vi "SV RMS Average Spectra (Complex).vi"(0 "complex spectra":T7(array[cluster]) {"spectrum info"."x-axis units" items=["Time (s)"=0, "Frequency-CB (Hz)"=1, "Frequency-CPB (Hz)"=1248, "Frequency-Arbitrary (Hz)"=2357, "Quefrency (s)"=2, "Revolutions (rev)"=3, "Order"=4, "Speed (RPM)"=11, "Speed (rad/s)"=21, "Index"=65535]; "spectrum info"."weighting filter" items=["Linear", "A-weighting", "B-weighting", "C-weighting", "ITU-R 468-4", "Dolby", "CCITT", "C-message", "Wb", "Wc", "Wd", "We", "Wf", "Wh", "Wj", "Wk", "Wm", "AES17 20 kHz lowpass", "AES17 40 kHz lowpass", "AES17 20 kHz highpass", "AES17 40 kHz highpass"]; "spectrum info"."dB reference [EU]" format="%.2f"; "spectrum info"."engineering units" items=["custom..."=0, "V"=1, "A"=21, "C"=30, "pC"=31, "s"=32, "-"=29, "Pa"=2, "N"=20, "g"=3, "m/s^2"=4, "m/s"=5, "m"=6, "mm/s"=12, "mm"=13, "micron/s"=14, "micron"=15, "in/s^2"=7, "in/s"=8, "in"=9, "mil/s"=10, "mil"=11, "rad/s^2"=16, "rad/s"=17, "rad"=18, "deg/s^2"=26, "deg/s"=27, "deg"=28, "RPM"=22, "cycle/s^2"=23, "Hz"=24, "cycle"=25, "strain"=19]; "spectrum info"."spectral info"."window" items=["None "=0, "Hanning"=1, "Hamming"=2, "Blackman-Harris"=3, "Exact Blackman"=4, "Blackman"=5, "Flat Top"=6, "4 Term B-Harris "=7, "7 Term B-Harris"=8, "Low Sidelobe"=9, "Force - Exponential"=10, "Gaussian"=62]; "complex spectrum response"."complex spectrum" format="%.2f"; "complex spectrum response"."df" format="%.2f"; "complex spectrum response"."f0" format="%.2f"}, 5 "error in (no error)":errorcluster) -> (13 "averages completed":dbl, 14 "rms average spectrum":cluster{"f0":dbl, "df":dbl, "magnitude":dbl[]} {"magnitude" format="%.2p"; "df" format="%.2p"; "f0" format="%.2p"}, 18 "spectrum info":T1={"channel name"="", "description"="", "x-axis units"=0, "spectral info"={"spectrum type"=enum."Power [Magnitude^2]", "linear/dB"=enum."linear", "window"=0, "window size"=0, "FFT size"=0}, "engineering units"=1, "custom label"="", "dB reference [EU]"=0.0, "peak units"=enum."rms", "weighting filter"=0, "spectral density?"=FALSE, "unit label"="", "spectrum skewed?"=FALSE, "complimentary spectrum units"=enum."none"} {"x-axis units" items=["Time (s)"=0, "Frequency-CB (Hz)"=1, "Frequency-CPB (Hz)"=1248, "Frequency-Arbitrary (Hz)"=2357, "Quefrency (s)"=2, "Revolutions (rev)"=3, "Order"=4, "Speed (RPM)"=11, "Speed (rad/s)"=21, "Index"=65535]; "weighting filter" items=["Linear", "A-weighting", "B-weighting", "C-weighting", "ITU-R 468-4", "Dolby", "CCITT", "C-message", "Wb", "Wc", "Wd", "We", "Wf", "Wh", "Wj", "Wk", "Wm", "AES17 20 kHz lowpass", "AES17 40 kHz lowpass", "AES17 20 kHz highpass", "AES17 40 kHz highpass"]; "dB reference [EU]" format="%.2f"; "engineering units" items=["custom..."=0, "V"=1, "A"=21, "C"=30, "pC"=31, "s"=32, "-"=29, "Pa"=2, "N"=20, "g"=3, "m/s^2"=4, "m/s"=5, "m"=6, "mm/s"=12, "mm"=13, "micron/s"=14, "micron"=15, "in/s^2"=7, "in/s"=8, "in"=9, "mil/s"=10, "mil"=11, "rad/s^2"=16, "rad/s"=17, "rad"=18, "deg/s^2"=26, "deg/s"=27, "deg"=28, "RPM"=22, "cycle/s^2"=23, "Hz"=24, "cycle"=25, "strain"=19]; "spectral info"."window" items=["None "=0, "Hanning"=1, "Hamming"=2, "Blackman-Harris"=3, "Exact Blackman"=4, "Blackman"=5, "Flat Top"=6, "4 Term B-Harris "=7, "7 Term B-Harris"=8, "Low Sidelobe"=9, "Force - Exponential"=10, "Gaussian"=62]}, 19 "error out":errorcluster)   [LabVIEW 2017]
doc: "Computes the linear RMS-averaged power spectrum of <B>scaled signal [EU]</B> in a linear scale. Use the power spectrum to quantify signal components as a function of frequency. Use this VI on embedded targets that have limited computational resources. Wire data to the <B>scaled signal [EU]</B> input to determine the polymorphic instance to use or manually select the instance."
uses:
  <vilib>/addons/_NISVFA/_Shared subVIs/Controls/svc_Spectrum Info.ctl
  <vilib>/addons/_NISVFA/_Shared subVIs/Controls/svc_X-Axis Units.ctl
  <vilib>/addons/_NISVFA/_Shared subVIs/Controls/svc_Spectrum Type.ctl
  <vilib>/addons/_NISVFA/_Shared subVIs/Controls/svc_Engineering Units Text Ring.ctl
  <vilib>/addons/_NISVFA/_Shared subVIs/Controls/svc_Weighting Filter Text Ring.ctl
  <vilib>/addons/_NISVFA/_Shared subVIs/Controls/svc_Complimentary Spectrum Units.ctl
  <vilib>/addons/_NISVFA/_Spectrum Processing/SVFA Unit Conversion (1 Ch).vi
  <vilib>/addons/_NISVFA/_Shared subVIs/Common/svc_Spectrum Units.vi
  <vilib>/addons/_NISVFA/_Spectrum Processing/subVIs/svfa_Conversion Utility (spectrum info).vi
  <vilib>/addons/_NISVFA/_Spectrum Processing/subVIs/svfa_Peak to RMS to Peak2Peak.vi
  <vilib>/addons/_NISVFA/_Spectrum Processing/subVIs/svfa_Mag to Mag2.vi
  <vilib>/addons/_NISVFA/_Spectrum Processing/subVIs/svfa_Linear to dB.vi
  <vilib>/addons/_NISVFA/_Spectrum Processing/subVIs/svfa_dBrefA to dBrefB.vi
  <vilib>/addons/_NISVFA/_Spectrum Processing/subVIs/svfa_Spectrum to Spectral Density.vi
  <vilib>/addons/_NISVFA/_Shared subVIs/Common/svc_Get Weighting Enum and Labels.vi
  <vilib>/addons/_NISVFA/_Shared subVIs/Common/svc_Unit Label Lexical Class.vi
  <vilib>/addons/_NISVFA/_Shared subVIs/Common/svc_Engineering Units to Unit Label.vi
  <vilib>/addons/_NISVFA/_Shared subVIs/Common/svc_Format Value (DBL).vi
  <vilib>/addons/_NISVFA/_Shared subVIs/Common/svc_Window Parameters.vi
  <vilib>/addons/_NISVFA/_Spectrum Processing/SVFA Unit Conversion (Complex) (1 Ch).vi
panel:
  out "unit label":string
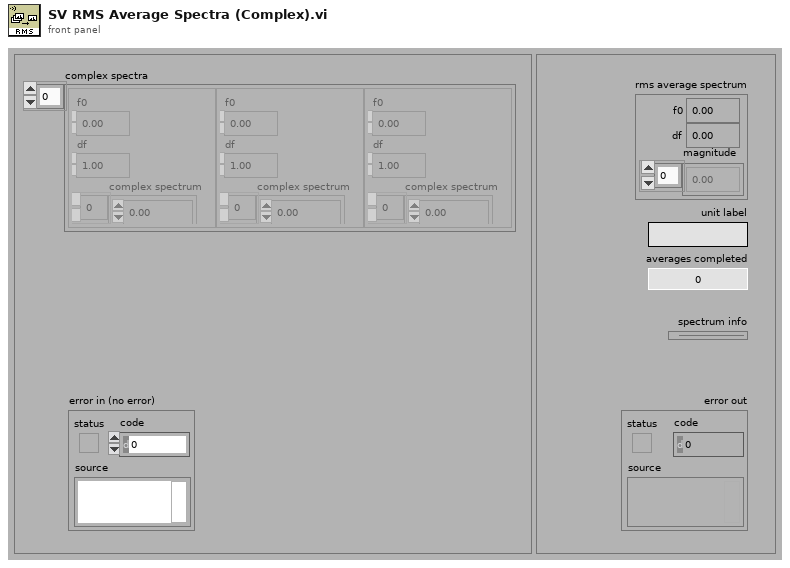
[diagram p1: front panel]
types:
  T1 = typedef "svc_Spectrum Info.ctl" = cluster{"channel name":string, "description":string, "x-axis units":T2, "spectral info":cluster{"spectrum type":T3, "linear/dB":enum16{"linear", "dB"}, "window":u16, "window size":i32, "FFT size":i32}, "engineering units":T4, "custom label":string, "dB reference [EU]":dbl, "peak units":enum16{"rms", "peak", "peak-peak"}, "weighting filter":T5, "spectral density?":bool, "unit label":string, "spectrum skewed?":bool, "complimentary spectrum units":T6}
  T2 = typedef "svc_X-Axis Units.ctl" = u16
  T3 = typedef "svc_Spectrum Type.ctl" = enum16{"FFT Spectrum [complex]", "Amplitude [Magnitude]", "Power [Magnitude^2]", "Cross Spectrum [complex]", "Frequency Response [Complex]"}
  T4 = typedef "svc_Engineering Units Text Ring.ctl" = u16
  T5 = typedef "svc_Weighting Filter Text Ring.ctl" = u16
  T6 = typedef "svc_Complimentary Spectrum Units.ctl" = enum16{"none", "radians", "degrees", "cycles", "imaginary"}
  T7 = cluster{"complex spectrum response":cluster{"f0":dbl, "df":dbl, "complex spectrum":cdb[]}, "spectrum info":T1}[]
  T8 = cluster{"linear/dB":enum16{"no change", "linear", "dB"}, "dB reference (0: no change)":dbl, "power/magnitude":enum16{"no change", "power", "magnitude"}, "view":enum16{"no change", "rms", "peak", "peak-peak"}}
  T9 = cluster{"complex spectrum response":cluster{"f0":dbl, "df":dbl, "complex spectrum":cdb[]}, "spectrum info":T1}
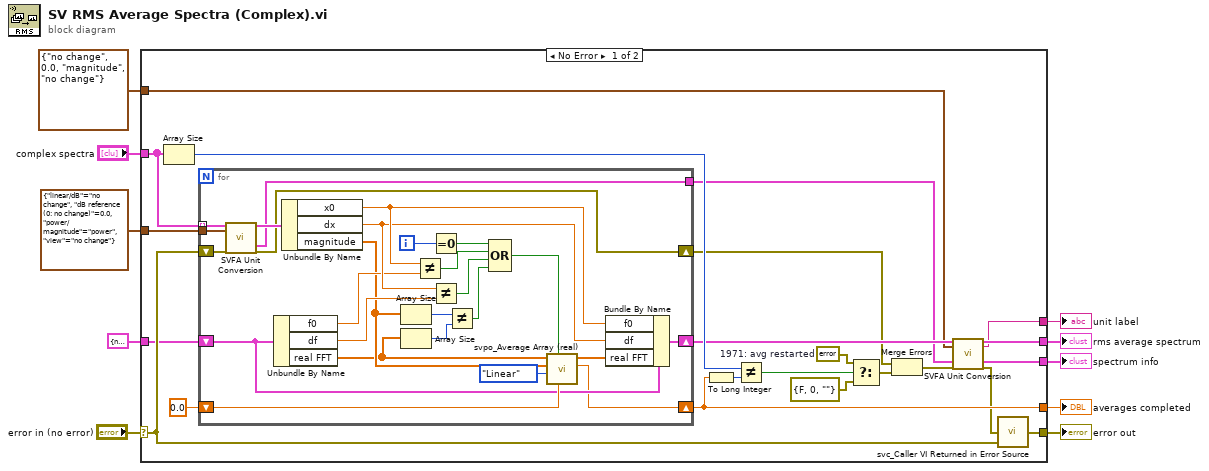
[diagram p0: block diagram]
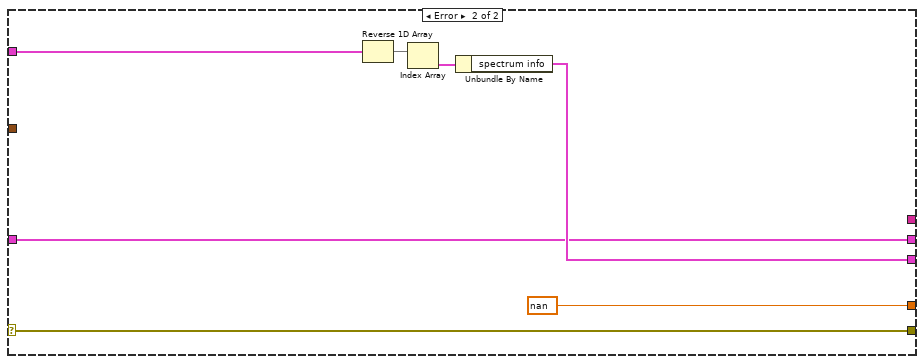
[diagram p2: hidden frame]
diagram:
  n1 = case shown="No Error" "error in (no error)" {
    selector: "error in (no error)" -> [w23 w64]
    tunnel: [w21 w59] -> w7
    tunnel: "complex spectra" -> [w24 w63]
    tunnel: [w31 nan ("Numeric")] -> w4
    tunnel: [w25 w64] -> w3
    tunnel: [w20 w60] -> w6
    tunnel: T8 {"linear/dB"=enum."no change", "dB reference (0: no change)"=0.0, "power/magnitude"=enum."power", "view"=enum."no change"} ("desired scaling") -> [w15 _]
    tunnel: [w14 _] -> w5
    tunnel: T8 {"linear/dB"=enum."no change", "dB reference (0: no change)"=0.0, "power/magnitude"=enum."magnitude", "view"=enum."no change"} ("desired scaling") -> [w12 _]
    tunnel: cluster{"f0":dbl, "df":dbl, "real FFT":dbl[]} {"f0"=nan, "df"=nan, "real FFT"=[]} ("previous avg real spectrum") -> [w11 w59]
    frame No Error {
      w28 = errorcluster {"status"=FALSE, "code"=1971, "source"="<append>\nAveraging restarted due to change in f0, df, or spectrum size within complex spectra input."}  # 1971: avg restarted
      n2 = Array Size(array=w24) -> (size(s)=w30:i32)
      n3 = for {
        tunnel: w24 -> [w36] mode=indexing
        shift-right: [w44] -> w31
        shift-left: 0.0 ("Numeric") -> [w52]
        shift-right: [w45] -> w22
        shift-left: w11 -> [w49]
        tunnel: w15 -> [w40]
        shift-right: [w38] -> w19
        shift-left: w23 -> [w39]
        tunnel: [w37] -> w16
        i -> [w50]
        n4 = call-poly <vilib>:"SVFA Unit Conversion.vi"("complex spectrum"=w36, "desired scaling"=w40, "error in (no error)"=w39) -> ("converted spectrum"=w41:cluster{"x0":dbl, "dx":dbl, "magnitude":dbl[]}, "spectrum info out"=w37:T1, "error out"=w38:errorcluster)  [unwired: 11 in, 3 out]
        n5 = Unbundle By Name(w49) -> ("f0"=w43:dbl, "df"=w42:dbl, "real FFT"=w33:dbl[])
        n6 = Unbundle By Name(w41) -> ("x0"=w47:dbl, "dx"=w46:dbl, "magnitude"=w34:dbl[])
        n7 = Array Size(array=w34) -> (size(s)=w58:i32)
        n8 = Array Size(array=w33) -> (size(s)=w57:i32)
        n9 = Not Equal?(x=w47, y=w43) -> (x != y?=w56:bool)
        n10 = Equal To 0?(x=w50) -> (x = 0?=w51:bool)
        n11 = Not Equal?(x=w46, y=w42) -> (x != y?=w54:bool)
        n12 = Not Equal?(x=w58, y=w57) -> (x != y?=w55:bool)
        n13 = Compound Arithmetic op=OR(w51, w56, w54, w55) -> (w35:bool)
        n14 = call <vilib>:"svpo_Average Array (real).vi"("averages completed in"=w52, "restart averaging"=w35, "weighting mode"=enum16{"Linear", "Exponential"}."Linear", "array"=w34, "previous average array"=w33) -> ("averages completed out"=w44:dbl, "average array"=w48:dbl[])  [unwired: 5 in]
        n15 = Bundle By Name(cluster=w49, "f0"=w47, "df"=w46, "real FFT"=w48) -> (w45:cluster{"f0":dbl, "df":dbl, "real FFT":dbl[]})
      }
      n16 = To Long Integer(number=w31) -> (32bit integer=w29:i32)
      n17 = Not Equal?(x=w30, y=w29) -> (x != y?=w26:bool)
      n18 = Select(t=w28, s=w26, f=errorcluster {"status"=FALSE, "code"=0, "source"=""}) -> (s? t:f=w18:errorcluster)
      n19 = Merge Errors(w19, w18) -> (w17:errorcluster)
      n20 = call-poly <vilib>:"SVFA Unit Conversion.vi"("spectrum"=w22, "desired scaling"=w12, "spectrum info in"=w16, "error in (no error)"=w17) -> ("converted spectrum"=w21:cluster{"x0":dbl, "dx":dbl, "magnitude":dbl[]}, "unit label"=w14:string, "spectrum info out"=w20:T1, "error out"=w13:errorcluster)  [unwired: 12 in]
      n21 = call <vilib>:"svc_Caller VI Returned in Error Source.vi"("warning input to caller"=w23, "error in (no error)"=w13) -> ("error out"=w25:errorcluster)  [unwired: 3 in]
    }
    frame Error {
      n22 = Reverse 1D Array(array=w63) -> (reversed array=w62:T7)
      n23 = Index Array(array=w62) -> (element=w61:T9)  [unwired: 1 in]
      n24 = Unbundle By Name(w61) -> ("spectrum info"=w60:T1)
    }
  }
  "rms average spectrum" <- w7
  "averages completed" <- w4
  "error out" <- w3
  "spectrum info" <- w6
  "unit label" <- w5
